vi "E12_BotonPulsador.vi"() -> ()   [LabVIEW 2026]
panel:
  in  "stop":bool
  out "Numeric":i32
  in  "Boolean":bool
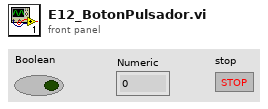
[diagram p1: front panel]
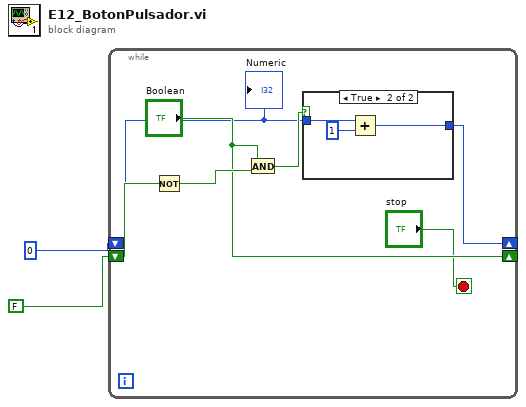
[diagram p0: block diagram]
diagram:
  n1 = while {
    shift-right: [w4] -> _
    shift-left: 0 -> [w5]
    shift-right: ["Boolean"] -> _
    shift-left: FALSE -> [w9]
    stop <- "stop" stop-if-true
    n2 = Not(x=w9) -> (.not. x?=w8:bool)
    n3 = And(x="Boolean", y=w8) -> (x .and. y?=w6:bool)
    n4 = case shown="True" w6 {
      tunnel: w5 -> [w10 w13]
      tunnel: [w10 w11] -> w4
      frame False {
      }
      frame True {
        n5 = Add(x=w13, y=1) -> (x+y=w11:i32)
      }
    }
    "Numeric" <- w5
  }
